vi "Scope Multi Records Panel.vi"() -> ()   [LabVIEW 2021]
doc: "Example: Multi Record\n\nRecommended Input Signal: 100 kHz, 8 Vpp, sine wave\n\nDevices Supported: Refer to NI Example Finders\n\nLabVIEW Description:\n\nThis VI demonstrates the multi-record capabilities of National Instruments high-speed oscilloscope. In a multi-record acquisition, each record is one waveform with at least \"min record length\" points as specified with the Configure Horizontal Timing VI. Furthermore, each record is triggered, so when the trigger arrives for the first record, the hardware quickly rearms for the next record. All records are stored in the onboard memory until they are retrieved with the Fetch VI. In this example, the Fetch VI has a positive timeout value, which pauses the program until all records have been acquired into the onboard memory before it fetches the waveforms.\n\nIf the \"plot relative to\" parameter is set to trigger, all records are overlaid on the same graph with the trigger occurring at time zero for each waveform. Notice that the points do not line up in time from different acquisitions. This is due to a very accurate measurement of the trigger time -- much more accurate than the time between two samples. The trigger time measurement is included in the relative initial x value, which is the time from the first sample to the trigger. It is returned by the Fetch VI. This accurate trigger time measurement is what allows random interleaved sampling to work. \n\nIf the \"plot relative to\" parameter is set to absolute, the records are all plotted on the same time scale. This feature is only available on oscilloscopes that support continuous acquisition. Using the absolute time scale, you will see the dead time, in which no points are acquired, between records. This allows you to compute the time between two records to the accuracy of the oscilloscope's sample clock. The absolute time is made possible by a free running, 48-bit counter on the oscilloscope. This counter is only cleared with the Reset, Abort, or Close VIs. Therefore, you could even use the absolute timestamp to compare the time between two software initiated acquisitions - the dead time would just be much longer. Refer to the NI High Speed Digitizers Help for more information about timestamps."
uses:
  <instrlib>/niScope/Configure/Trigger/niScope Configure Trigger Digital.vi
  <instrlib>/niScope/Configure/Trigger/niScope Configure Trigger Edge.vi
  <instrlib>/niScope/Configure/Trigger/niScope Configure Trigger Immediate.vi
  <instrlib>/niScope/Configure/Trigger/niScope Configure Trigger Hysteresis.vi
  <instrlib>/niScope/Configure/Trigger/niScope Configure Trigger Window.vi
  <instrlib>/niScope/Configure/niScope Import Attribute Configuration File.vi
  <instrlib>/niScope/Acquire/Fetch/niScope Multi Fetch.vi
  <instrlib>/niScope/Configure/niScope Export Attribute Configuration File.vi
panel:
  out "Final Configuration Buffer":string
  in  "Export Configuration After Finished?":bool
  out "Actual Sample Rate":dbl=10000000.0 step=1000000.0 format="%#.3p"
  out "Actual Record Length":i32=256 min=0
  in  "Timeout (s)":dbl=5.0 format="%#_6p"
  in  "Reference Position":dbl(slide)=50.0 caption="Ref Position (%)" min=0.0 max=100.0 step=5.0 scale=0.0..100.0
  in  "Config Method":enum32{"Manual", "Config File"}(tab)
  in  "Vertical Range (V)":dbl=5.0 format="%#.2p"
  in  "Min. Sample Rate":dbl=10000000.0 step=1000000.0 format="%#.3p"
  in  "Trigger Type":T1(tab)
  in  "Edge Trigger":T2={"Trigger Coupling"=1, "Trigger Slope"=0, "Trigger Level"=0.0, "Trigger Source"="0"} {"Trigger Level" format="%.2f"; "Trigger Slope" items=["Positive", "Negative"]; "Trigger Coupling" items=["AC"=0, "DC"=1, "HF Reject"=3, "LF Reject"=4, "AC Plus HF Reject"=1001]}
  in  "Digital Trigger":T3={"Trigger Source"="VAL_PFI_1", "Trigger Slope"=0} {"Trigger Slope" items=["Positive", "Negative"]}
  in  "Window Trigger":T4={"Trigger Source"="0", "Window Mode"=0, "Window Low Level"=-0.1, "Window High Level"=0.1, "Trigger Coupling"=1} {"Trigger Coupling" items=["AC"=0, "DC"=1, "HF Reject"=3, "LF Reject"=4, "AC Plus HF Reject"=1001]; "Window High Level" format="%.2f"; "Window Low Level" format="%.2f"; "Window Mode" items=["Entering", "Leaving"]}
  in  "Hysteresis Trigger":T5={"Trigger Slope"=0, "Trigger Coupling"=1, "Trigger Level"=0.0, "Trigger Source"="0", "Hysteresis"=0.05} {"Hysteresis" format="%.2f"; "Trigger Level" format="%.2f"; "Trigger Coupling" items=["AC"=0, "DC"=1, "HF Reject"=3, "LF Reject"=4, "AC Plus HF Reject"=1001]; "Trigger Slope" items=["Positive", "Negative"]}
  in  "Min. Record Length":i32=256 min=0
  in  "Configuration File Path":path
  out "Waveform Graph":T6(graph)
  in  "Number Of Records":i32=2 min=1 step=1
  in  "Channel Name":string="0"
  in  "Resource Name":refnum<k15>="Dev1" caption="Resource Name(s)"
  # "NI Scope Multi Records Panel"
  # "Right-click the graph to export waveforms to file"
  # "Note: When configured for Immediate reference trigger, this example does not configure any additional trigger settings - the acquisition is triggered as soon as possible after being initiated by driver software."
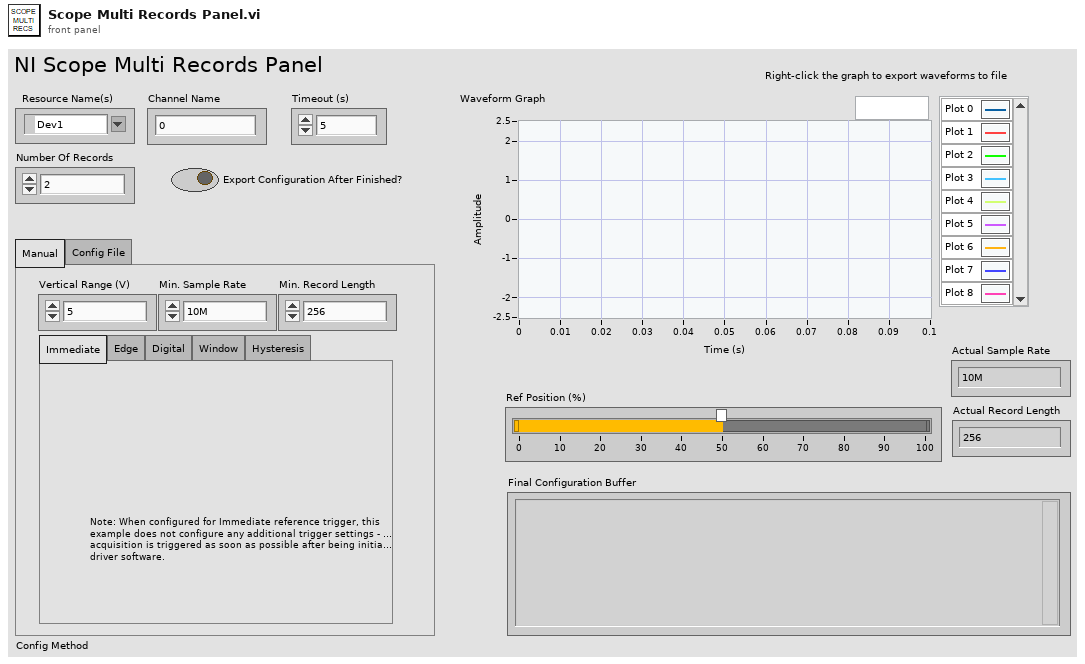
[diagram p1: front panel]
types:
  T1 = enum32{"Immediate", "Edge", "Digital", "Window", "Hysteresis"}
  T2 = cluster{"Trigger Coupling":u16, "Trigger Slope":i32, "Trigger Level":dbl, "Trigger Source":string}
  T3 = cluster{"Trigger Source":string, "Trigger Slope":i32}
  T4 = cluster{"Trigger Source":string, "Window Mode":i32, "Window Low Level":dbl, "Window High Level":dbl, "Trigger Coupling":u16}
  T5 = cluster{"Trigger Slope":i32, "Trigger Coupling":u16, "Trigger Level":dbl, "Trigger Source":string, "Hysteresis":dbl}
  T6 = cluster{"relativeInitialX":dbl, "xIncrement":dbl, "wfm":dbl[]}[]
  T7 = cluster{"actualSamples":i32, "absoluteInitialX":dbl, "relativeInitialX":dbl, "xIncrement":dbl, "offset":dbl, "gain":dbl, "reserved1":dbl, "reserved2":dbl}[]
  T8 = cluster{"relativeInitialX":dbl, "xIncrement":dbl, "wfm":dbl[]}
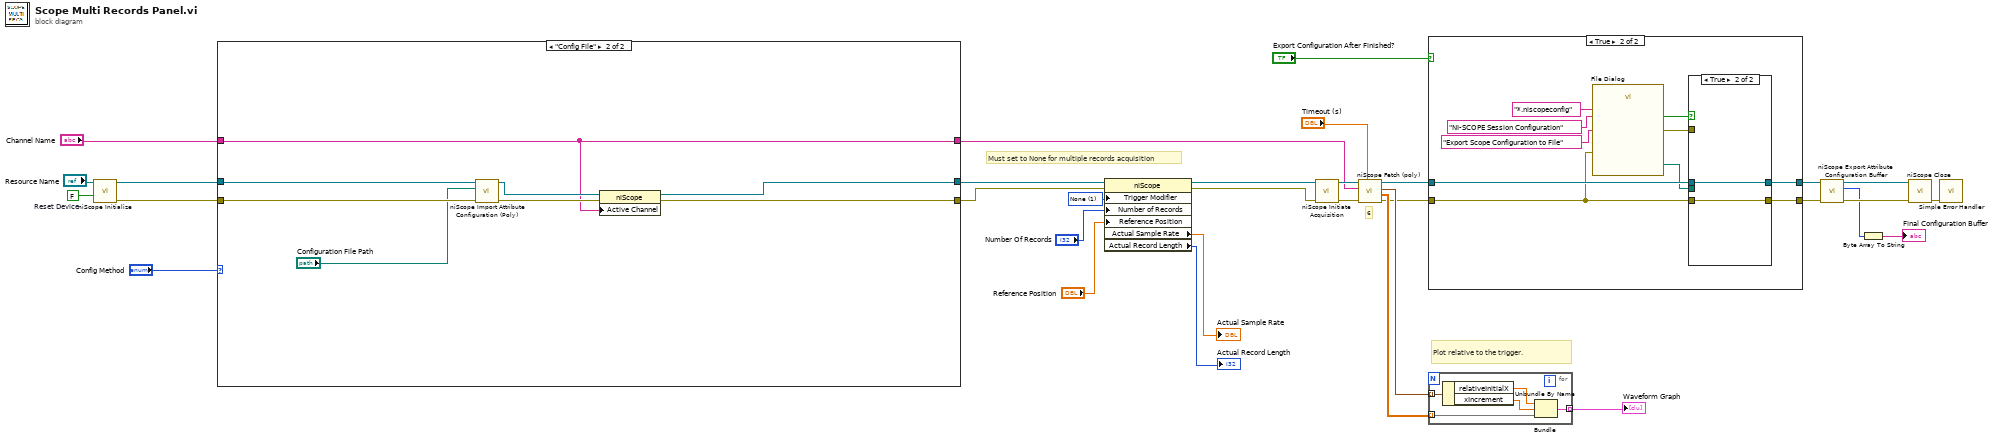
[diagram p0: block diagram]
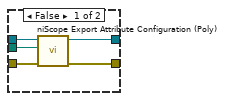
[diagram p3: hidden frame]
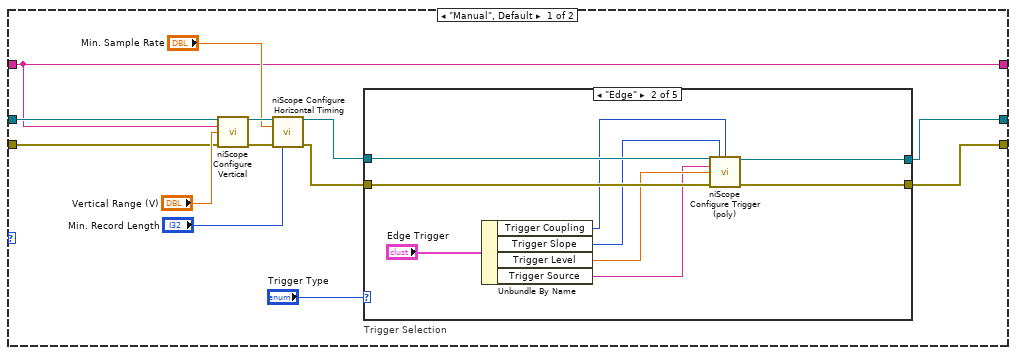
[diagram p4: hidden frame]
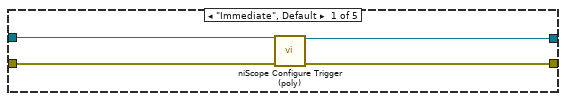
[diagram p5: hidden frame]
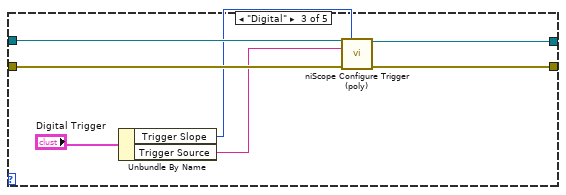
[diagram p6: hidden frame]
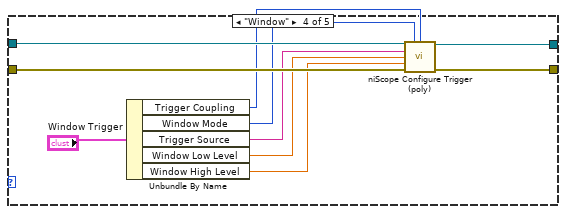
[diagram p7: hidden frame]
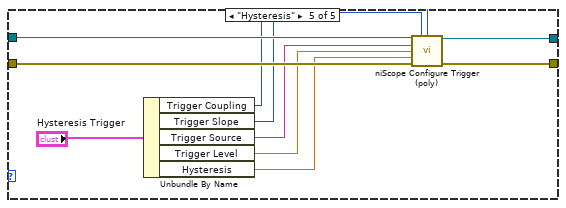
[diagram p8: hidden frame]
diagram:
  w1 = 1 items=["None"=1, "Auto Trigger"=2] ("Triggering:Trigger Modifier")
  w32 = FALSE  # Reset Device
  # "Must set to None for multiple records acquisition"
  # "Plot relative to the trigger."
  # "6"
  n1 = call <instrlib>:"niScope Initialize.vi"("resource name"="Resource Name", "reset device"=w32) -> ("instrument handle"=w30:refnum<k15>, "error out"=w29:errorcluster)  [unwired: 12 in]
  n2 = case shown="\"Config File\"" "Config Method" {
    tunnel: w30 -> [w40 w91]
    tunnel: w29 -> [w39 w93]
    tunnel: [w35 w87] -> w17
    tunnel: [w34 w89] -> w26
    tunnel: "Channel Name" -> [w38 w86]
    tunnel: [w38 w86] -> w19
    frame "Manual", Default {
      n3 = call <instrlib>:"niScope Configure Vertical.vi"("instrument handle"=w40, "channels"=w38, "vertical range"="Vertical Range (V)", "error in"=w39) -> ("instrument handle out"=w44:refnum<k15>, "error out"=w45:errorcluster)  [unwired: 10 in]
      n4 = call <instrlib>:"niScope Configure Horizontal Timing.vi"("instrument handle"=w44, "min sample rate"="Min. Sample Rate", "error in"=w45, "min record length"="Min. Record Length") -> ("instrument handle out"=w37:refnum<k15>, "error out"=w36:errorcluster)  [unwired: 10 in]
      n5 = case "Trigger Selection" shown="\"Edge\"" "Trigger Type" {
        tunnel: w36 -> [w49 w58 w65 w75 w85]
        tunnel: [w46 w55 w62 w72 w82] -> w34
        tunnel: w37 -> [w48 w57 w64 w74 w84]
        tunnel: [w47 w56 w63 w73 w83] -> w35
        frame "Immediate", Default {
          n6 = call-poly <instrlib>:"niScope Configure Trigger (poly).vi"("instrument handle"=w48, "error in"=w49) -> ("instrument handle out"=w47:refnum<k15>, "error out"=w46:errorcluster)  [unwired: 12 in]
        }
        frame "Edge" {
          n7 = Unbundle By Name("Edge Trigger") -> ("Trigger Coupling"=w53:u16, "Trigger Slope"=w52:i32, "Trigger Level"=w51:dbl, "Trigger Source"=w50:string)
          n8 = call-poly <instrlib>:"niScope Configure Trigger (poly).vi"("instrument handle"=w57, "trigger slope"=w52, "trigger coupling"=w53, "trigger source"=w50, "trigger level"=w51, "error in"=w58) -> ("instrument handle out"=w56:refnum<k15>, "error out"=w55:errorcluster)  [unwired: 8 in]
        }
        frame "Digital" {
          n9 = Unbundle By Name("Digital Trigger") -> ("Trigger Slope"=w60:i32, "Trigger Source"=w59:string)
          n10 = call-poly <instrlib>:"niScope Configure Trigger (poly).vi"("instrument handle"=w64, "trigger slope"=w60, "trigger source"=w59, "error in"=w65) -> ("instrument handle out"=w63:refnum<k15>, "error out"=w62:errorcluster)  [unwired: 10 in]
        }
        frame "Window" {
          n11 = Unbundle By Name("Window Trigger") -> ("Trigger Coupling"=w70:u16, "Window Mode"=w69:i32, "Trigger Source"=w68:string, "Window Low Level"=w67:dbl, "Window High Level"=w66:dbl)
          n12 = call-poly <instrlib>:"niScope Configure Trigger (poly).vi"("instrument handle"=w74, "trigger window mode"=w69, "trigger coupling"=w70, "trigger source"=w68, "low level"=w67, "high level"=w66, "error in"=w75) -> ("instrument handle out"=w73:refnum<k15>, "error out"=w72:errorcluster)  [unwired: 7 in]
        }
        frame "Hysteresis" {
          n13 = Unbundle By Name("Hysteresis Trigger") -> ("Trigger Coupling"=w80:u16, "Trigger Slope"=w79:i32, "Trigger Source"=w78:string, "Trigger Level"=w77:dbl, "Hysteresis"=w76:dbl)
          n14 = call-poly <instrlib>:"niScope Configure Trigger (poly).vi"("instrument handle"=w84, "trigger slope"=w79, "trigger coupling"=w80, "trigger source"=w78, "trigger level"=w77, "hysteresis"=w76, "error in"=w85) -> ("instrument handle out"=w83:refnum<k15>, "error out"=w82:errorcluster)  [unwired: 7 in]
        }
      }
    }
    frame "Config File" {
      n15 = call-poly <instrlib>:"niScope Import Attribute Configuration (Poly).vi"("error in"=w93, "file path"="Configuration File Path", "instrument handle"=w91) -> ("error out"=w92:errorcluster, "instrument handle out"=w88:refnum<k15>)  [unwired: 7 in]
      n16 = property class="niScope"(reference=w88, error in=w92, "Active Channel"=w86) -> (reference out=w87:refnum<k15>, error out=w89:errorcluster)
    }
  }
  n17 = property class="niScope"(reference=w17, error in=w26, "Trigger Modifier"=w1, "Number of Records"="Number Of Records", "Reference Position"="Reference Position") -> (reference out=w16:refnum<k15>, error out=w18:errorcluster, "Actual Sample Rate"=→"Actual Sample Rate":dbl, "Actual Record Length"=→"Actual Record Length":i32)
  n18 = call <instrlib>:"niScope Initiate Acquisition.vi"("instrument handle"=w16, "error in"=w18) -> ("instrument handle out"=w24:refnum<k15>, "error out"=w25:errorcluster)  [unwired: 12 in]
  n19 = call-poly <instrlib>:"niScope Fetch (poly).vi"("timeout"="Timeout (s)", "error in"=w25, "channels"=w19, "instrument handle"=w24) -> ("error out"=w22:errorcluster, "wfm"=w28:dbl[][], "wfm info"=w27:T7, "instrument handle out"=w9:refnum<k15>)  [unwired: 4 in]
  n20 = case shown="True" "Export Configuration After Finished?" {
    tunnel: w22 -> [w94 w96]
    tunnel: [w94 w105] -> w10
    tunnel: w9 -> [w95 w104]
    tunnel: [w95 w103] -> w6
    frame False {
    }
    frame True {
      n21 = call "File Dialog"("prompt"="Export Scope Configuration to File", "error in"=w96, "pattern (all files)"="*.niscopeconfig", "pattern label"="NI-SCOPE Session Configuration") -> ("selected path"=w99:path, "cancelled"=w98:bool, "error out"=w97:errorcluster)  [unwired: 8 in, 1 out]
      n22 = case shown="True" w98 {
        tunnel: w96 -> [w110 w111]
        tunnel: [w109 w111] -> w105
        tunnel: w104 -> [w108 w112]
        tunnel: [w107 w112] -> w103
        tunnel: w99 -> [w106 _]
        tunnel: w97 -> [_ _]
        frame False {
          n23 = call-poly <instrlib>:"niScope Export Attribute Configuration (Poly).vi"("error in"=w110, "file path"=w106, "instrument handle"=w108) -> ("error out"=w109:errorcluster, "instrument handle out"=w107:refnum<k15>)  [unwired: 7 in]
        }
        frame True {
        }
      }
    }
  }
  n24 = for {
    tunnel: w28 -> [w115] mode=indexing
    tunnel: [w114] -> w20 mode=indexing
    tunnel: w27 -> [w113] mode=indexing
    n25 = Unbundle By Name(w113) -> ("relativeInitialX"=w117:dbl, "xIncrement"=w116:dbl)
    n26 = Bundle("relativeInitialX"=w117, "xIncrement"=w116, "wfm"=w115) -> (w114:T8)  [unwired: 1 in]
  }
  "Waveform Graph" <- w20
  n27 = call <instrlib>:"niScope Export Attribute Configuration Buffer.vi"("error in"=w10, "instrument handle"=w6) -> ("error out"=w7:errorcluster, "buffer"=w4:u8[], "instrument handle out"=w5:refnum<k15>)  [unwired: 7 in]
  n28 = Byte Array To String(unsigned byte array=w4) -> (string=→"Final Configuration Buffer":string)
  n29 = call <instrlib>:"niScope Close.vi"("instrument handle"=w5, "error in"=w7) -> ("error out"=w23:errorcluster)  [unwired: 13 in]
  n30 = call <vilib>:"Simple Error Handler.vi"("error in (no error)"=w23) -> ()  [unwired: 4 in, 5 out]
